vi "Begin.vi"() -> (0 "error out":errorcluster)   [LabVIEW 2012]
doc: "Called before other user functions, this VI is expected to open initial I/O refnums, load in file data, and do all program initialization. Notice that the <B>error out</B> terminal is simply used for data flow. Wiring it to other structures or subVIs ensures that this VI runs first."
uses:
  <vilib>/Rock Robotics/WPI/DriverStation/WPI_DriverStationRobotMode2.ctl
  <vilib>/Rock Robotics/WPI/CAN/Jaguar/SubVIs/WPI_CANJaguar_ControlMode.ctl
  <vilib>/Rock Robotics/WPI/CAN/Jaguar/SubVIs/WPI_CANJaguar_PositionReference.ctl
  <vilib>/Rock Robotics/WPI/CAN/Jaguar/SubVIs/WPI_CANJaguar_BrakeCoastMode.ctl
  <vilib>/Rock Robotics/WPI/SafetyOutput/WPI_SafetyOutputConfigMenu.ctl
  <vilib>/Rock Robotics/SystemInterfaces/DIO/FPGA_DIOChannel.ctl
  <vilib>/Rock Robotics/SystemInterfaces/DIO/FPGA_DIOPWMChannel.ctl
  <vilib>/Rock Robotics/WPI/CAN/Jaguar/SubVIs/WPI_CANJaguar_SpeedReference.ctl
  <vilib>/Rock Robotics/WPI/Joystick/WPI_JoystickDeviceEnum.ctl
  Robot Global Data.vi
  <vilib>/Rock Robotics/WPI/MotorControl/WPI_MotorControlOpenCANJaguar.vi
  <vilib>/Rock Robotics/WPI/MotorControl/WPI_MotorControlOpen Victor.vi
  <vilib>/Rock Robotics/WPI/RobotDrive/WPI_RobotDriveOpen4MotorWithExistingMotors.vi
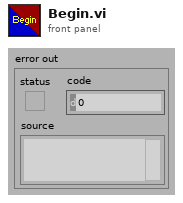
[diagram p1: front panel]
types:
  T1 = typedef "WPI_DriverStationRobotMode2.ctl" = enum16{"Autonomous Disabled", "Autonomous Enabled", "Teleop Disabled", "Teleop Enabled", "Timeout", "Finish", "Test Disabled", "Test Enabled"}
  T2 = typedef "WPI_CANJaguar_BrakeCoastMode.ctl" = enum8{"Jumper", "Brake", "Coast"}
  T3 = typedef "WPI_CANJaguar_ControlMode.ctl" = enum8{"Percent VBus", "Current", "Speed", "Position", "Voltage"}
  T4 = typedef "WPI_MotorControlDeviceRef.ctl" = cluster{"DeviceStatus":errorcluster, "Type":enum16{"PWM", "CAN"}, "PWM":cluster{"Digital Module":T5, "PWM Channel":T6, "DeadBand":T7}, "CAN":cluster{"Device Number":u8, "Control Mode":T3, "Semaphore":T8, "Max Vout":dbl}, "Invert":bool, "TransformRef":T9, "InvTransformRef":T9}
  T5 = typedef "FPGA_TypedefDigitalModule.ctl" = enum16{"Digital Module 1", "Digital Module 2"}
  T6 = typedef "FPGA_DIOPWMChannel.ctl" = enum8{"PWM 1", "PWM 2", "PWM 3", "PWM 4", "PWM 5", "PWM 6", "PWM 7", "PWM 8", "PWM 9", "PWM 10", "Invalid"}
  T7 = typedef "WPI_PWMDeadband.ctl" = cluster{"Name":string, "maxPositivePwm":i32, "minPositivePwm":i32, "centerPwm":i32, "maxNegativePwm":i32, "minNegativePwm":i32, "angularRange":u16}
  T8 = typedef "Semaphore RefNum" = refnum<k1>
  T9 = typedef "WPI_PWMTransform_ConPane.ctl" = refnum<vi>
  T10 = typedef "WPI_CANJaguar_SpeedReference.ctl" = u8
  T11 = typedef "WPI_RobotDriveDevRef.ctl" = cluster{"DevStatus":errorcluster, "Motors[]":T4[], "Square Inputs":bool, "Max Output":dbl, "Isochronous":bool}
  T12 = typedef "WPI_SafetyOutputConfigMenu.ctl" = enum16{"Enable", "Disable"}
  T13 = typedef "WPI_CANJaguar_PositionReference.ctl" = u8
  T14 = typedef "WPI_JoystickDeviceEnum.ctl" = enum16{"USB 1", "USB 2", "USB 3", "USB 4", "Kinect 1", "Kinect 2"}
  T15 = typedef "WPI_JoystickDevRef.ctl" = cluster{"Device":T14}
  T16 = typedef "FPGA_DIOChannel.ctl" = enum8{"DIO 1", "DIO 2", "DIO 3", "DIO 4", "DIO 5", "DIO 6", "DIO 7", "DIO 8", "DIO 9", "DIO 10", "DIO 11", "DIO 12", "DIO 13", "DIO 14", "Invalid"}
  T17 = typedef "WPI_DigitalInputDevRef.ctl" = cluster{"DevStatus":errorcluster, "DIO Channel":T16, "Digital Module":T5}
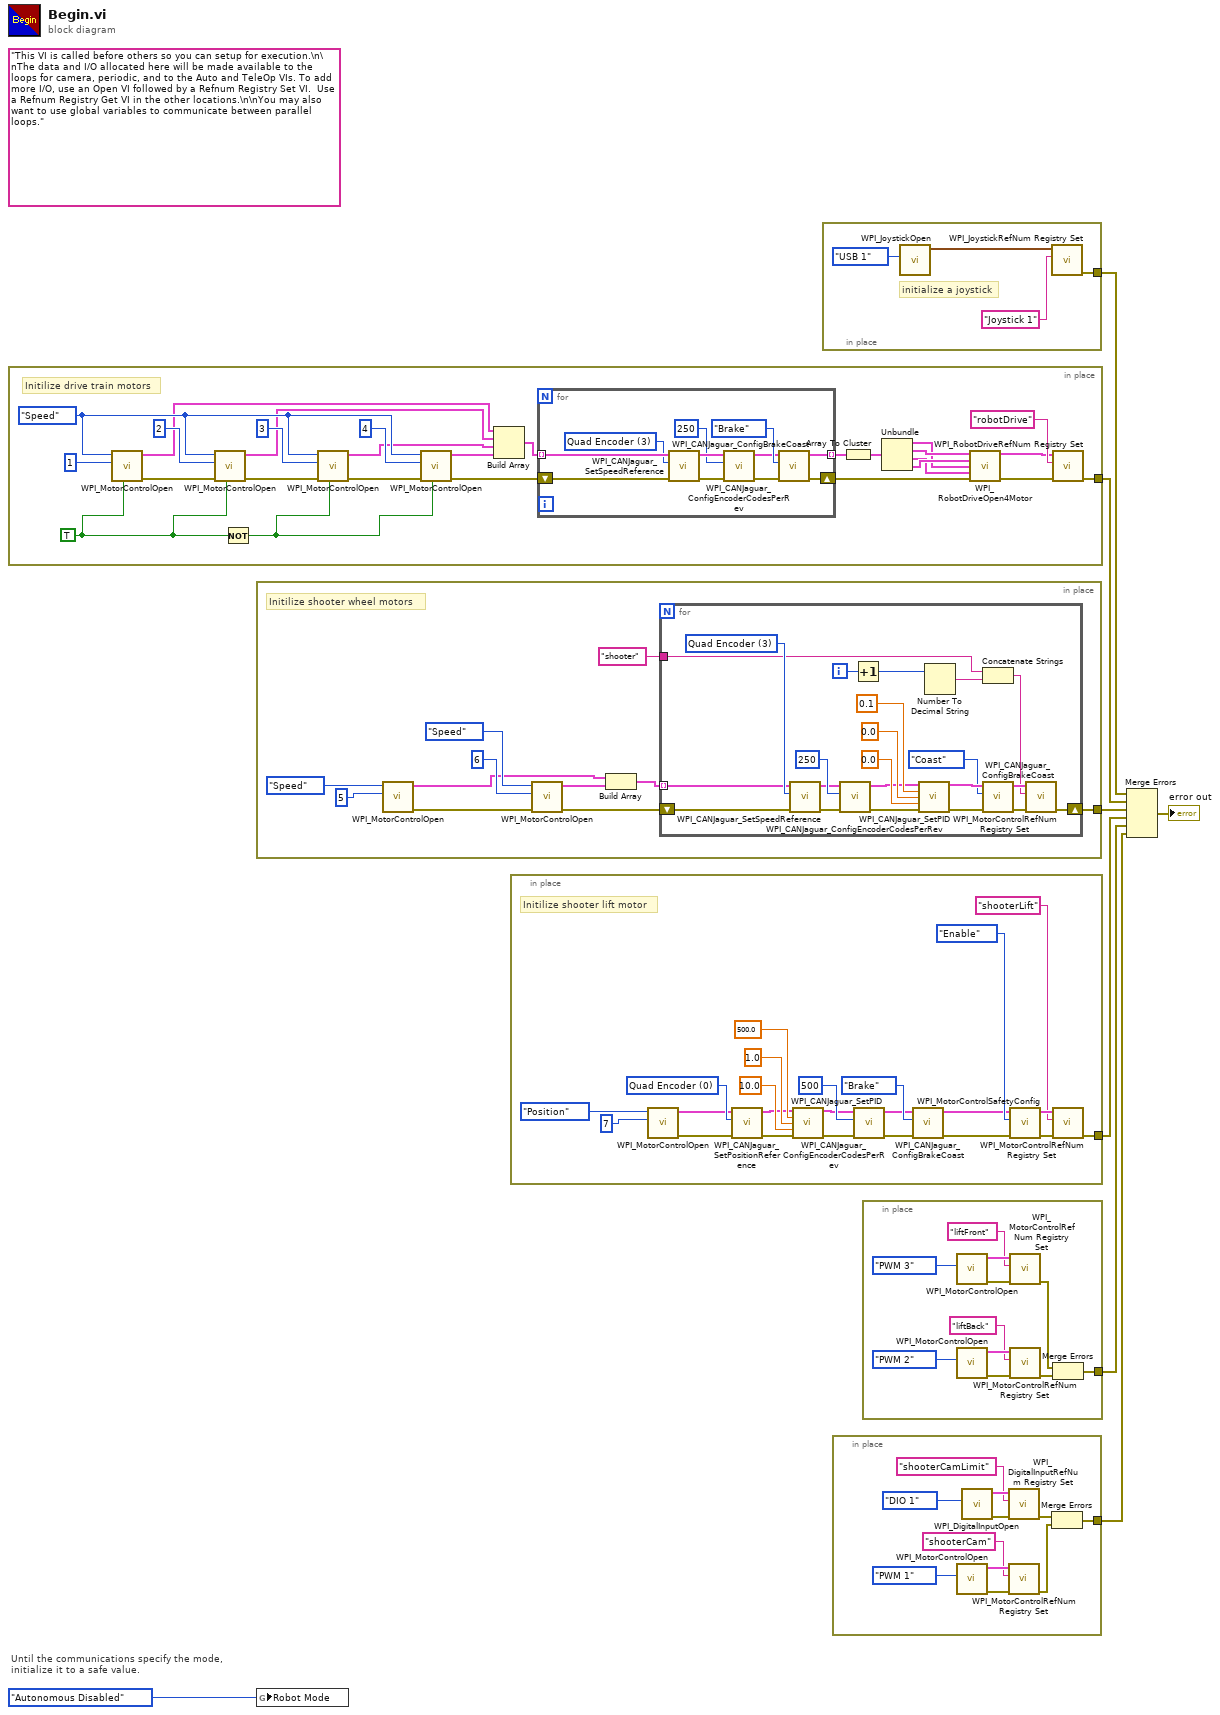
[diagram p0: block diagram]
diagram:
  (unwired) "This VI is called before others so you can setup for execution.\n\nThe data and I/O allocated here will be made available to the loops for camera, periodic, and to the Auto and TeleOp VIs. To add more I/O, use an Open VI followed by a Refnum Registry Set VI.  Use a Refnum Registry Get VI in the other locations.\n\nYou may also want to use global variables to communicate between parallel loops."
  # "Until the communications specify the mode,\ninitialize it to a safe value."
  n1 = in-place {
    in-place-border: [w35] -> w7
    w29 = TRUE ("Invert")
    w34 = WPI_CANJaguar_ControlMode."Speed" ("Control Mode")
    # "Initilize drive train motors"
    n2 = call-poly <vilib>:"WPI_MotorControlOpen.vi"("Invert"=w29, "Device Number"=u8 1, "Control Mode"=w34) -> ("error out"=w27:errorcluster, "MotorControlDeviceRef"=w24:T4)  [unwired: 7 in]
    n3 = call-poly <vilib>:"WPI_MotorControlOpen.vi"("Invert"=w29, "error in (no error)"=w27, "Device Number"=u8 2, "Control Mode"=w34) -> ("error out"=w26:errorcluster, "MotorControlDeviceRef"=w23:T4)  [unwired: 6 in]
    n4 = Not(x=w29) -> (.not. x?=w28:bool)
    n5 = call-poly <vilib>:"WPI_MotorControlOpen.vi"("Invert"=w28, "error in (no error)"=w26, "Device Number"=u8 3, "Control Mode"=w34) -> ("error out"=w25:errorcluster, "MotorControlDeviceRef"=w22:T4)  [unwired: 6 in]
    n6 = call-poly <vilib>:"WPI_MotorControlOpen.vi"("Invert"=w28, "error in (no error)"=w25, "Device Number"=u8 4, "Control Mode"=w34) -> ("error out"=w10:errorcluster, "MotorControlDeviceRef"=w21:T4)  [unwired: 6 in]
    n7 = Build Array(w24, w23, w22, w21) -> (w19:T4[])
    n8 = for {
      tunnel: w19 -> [w43] mode=indexing
      tunnel: [w45] -> w18 mode=indexing
      shift-right: [w44] -> w9
      shift-left: w10 -> [w42]
      w41 = T10 3 items=["Encoder"=0, "Inv Encoder"=2, "Quad Encoder"=3, "None"=255] ("Speed Reference")
      n9 = call <vilib>:"WPI_CANJaguar_SetSpeedReference.vi"("error in (no error)"=w42, "Speed Reference"=w41, "CAN Jaguar Ref"=w43) -> ("error out"=w40:errorcluster, "CAN Jaguar Ref Out"=w39:T4)  [unwired: 7 in]
      n10 = call <vilib>:"WPI_CANJaguar_ConfigEncoderCodesPerRev.vi"("error in (no error)"=w40, "Encoder Codes Per Rev"=u16 250, "CAN Jaguar Ref"=w39) -> ("error out"=w36:errorcluster, "CAN Jaguar Ref Out"=w37:T4)  [unwired: 7 in]
      n11 = call <vilib>:"WPI_CANJaguar_ConfigBrakeCoast.vi"("error in (no error)"=w36, "Brake / Coast Mode"=WPI_CANJaguar_BrakeCoastMode."Brake", "CAN Jaguar Ref"=w37) -> ("error out"=w44:errorcluster, "CAN Jaguar Ref Out"=w45:T4)  [unwired: 7 in]
    }
    n12 = Array To Cluster(array=w18) -> (cluster=w17:cluster{"[0]":T4, "[1]":T4, "[2]":T4, "[3]":T4})
    n13 = Unbundle(w17) -> ("[0]"=w11:T4, "[1]"=w12:T4, "[2]"=w13:T4, "[3]"=w14:T4)
    n14 = call-poly <vilib>:"WPI_RobotDriveOpen4Motor.vi"("Rear Left Motor Dev Ref"=w12, "Rear Right Motor Dev Ref"=w14, "Front Left Motor Dev Ref"=w11, "Front Right Motor Dev Ref"=w13, "error in (no error)"=w9) -> ("RobotDriveDevRef"=w15:T11, "error out"=w16:errorcluster)  [unwired: 9 in]
    n15 = call <vilib>:"WPI_RobotDriveRefNum Registry Set.vi"("error in (no error)"=w16, "refnum name"="robotDrive", "RobotDriveDevRef"=w15) -> ("error out"=w35:errorcluster)  [unwired: 7 in, 1 out]
  }
  n16 = in-place {
    in-place-border: [w57] -> w6
    # "Initilize shooter wheel motors"
    n17 = call-poly <vilib>:"WPI_MotorControlOpen.vi"("Device Number"=u8 5, "Control Mode"=WPI_CANJaguar_ControlMode."Speed") -> ("error out"=w52:errorcluster, "MotorControlDeviceRef"=w50:T4)  [unwired: 8 in]
    n18 = call-poly <vilib>:"WPI_MotorControlOpen.vi"("error in (no error)"=w52, "Device Number"=u8 6, "Control Mode"=WPI_CANJaguar_ControlMode."Speed") -> ("error out"=w48:errorcluster, "MotorControlDeviceRef"=w51:T4)  [unwired: 7 in]
    n19 = Build Array(w50, w51) -> (w49:T4[])
    n20 = for {
      tunnel: w49 -> [w68] mode=indexing
      tunnel: "shooter" -> [w62]
      shift-right: [w59] -> w57
      shift-left: w48 -> [w67]
      i -> [w66]
      w69 = T10 3 items=["Encoder"=0, "Inv Encoder"=2, "Quad Encoder"=3, "None"=255] ("Speed Reference")
      n21 = call <vilib>:"WPI_CANJaguar_SetSpeedReference.vi"("error in (no error)"=w67, "Speed Reference"=w69, "CAN Jaguar Ref"=w68) -> ("error out"=w70:errorcluster, "CAN Jaguar Ref Out"=w71:T4)  [unwired: 7 in]
      n22 = call <vilib>:"WPI_CANJaguar_ConfigEncoderCodesPerRev.vi"("error in (no error)"=w70, "Encoder Codes Per Rev"=u16 250, "CAN Jaguar Ref"=w71) -> ("error out"=w74:errorcluster, "CAN Jaguar Ref Out"=w73:T4)  [unwired: 7 in]
      n23 = Increment(x=w66) -> (x+1=w65:i32)
      n24 = call <vilib>:"WPI_CANJaguar_SetPID.vi"("CAN Jaguar Ref"=w73, "P"=0.1, "I"=0.0, "D"=0.0, "error in (no error)"=w74) -> ("CAN Jaguar Ref Out"=w75:T4, "error out"=w76:errorcluster)  [unwired: 9 in]
      n25 = Number To Decimal String(number=w65) -> (decimal integer string=w61:string)  [unwired: 1 in]
      n26 = Concatenate Strings(w62, w61) -> (w60:string)
      n27 = call <vilib>:"WPI_CANJaguar_ConfigBrakeCoast.vi"("error in (no error)"=w76, "Brake / Coast Mode"=WPI_CANJaguar_BrakeCoastMode."Coast", "CAN Jaguar Ref"=w75) -> ("error out"=w64:errorcluster, "CAN Jaguar Ref Out"=w63:T4)  [unwired: 7 in]
      n28 = call <vilib>:"WPI_MotorControlRefNum Registry Set.vi"("error in (no error)"=w64, "refnum name"=w60, "MotorControlDevRef"=w63) -> ("error out"=w59:errorcluster)  [unwired: 7 in, 1 out]
    }
  }
  n29 = global write "Robot Global Data.vi" "Robot Mode"(WPI_DriverStationRobotMode2."Autonomous Disabled" ("Robot Mode")) -> ()
  n30 = in-place {
    in-place-border: [w102] -> w3
    w88 = T13 0 items=["Quad Encoder"=0, "Potentiometer"=1, "None"=255] ("Position Reference")
    # "Initilize shooter lift motor"
    n31 = call-poly <vilib>:"WPI_MotorControlOpen.vi"("Device Number"=u8 7, "Control Mode"=WPI_CANJaguar_ControlMode."Position") -> ("error out"=w86:errorcluster, "MotorControlDeviceRef"=w87:T4)  [unwired: 8 in]
    n32 = call <vilib>:"WPI_CANJaguar_SetPositionReference.vi"("error in (no error)"=w86, "Position Reference"=w88, "CAN Jaguar Ref"=w87) -> ("error out"=w90:errorcluster, "CAN Jaguar Ref Out"=w89:T4)  [unwired: 7 in]
    n33 = call <vilib>:"WPI_CANJaguar_SetPID.vi"("CAN Jaguar Ref"=w89, "P"=500.0, "I"=1.0, "D"=10.0, "error in (no error)"=w90) -> ("CAN Jaguar Ref Out"=w95:T4, "error out"=w94:errorcluster)  [unwired: 9 in]
    n34 = call <vilib>:"WPI_CANJaguar_ConfigEncoderCodesPerRev.vi"("error in (no error)"=w94, "Encoder Codes Per Rev"=u16 500, "CAN Jaguar Ref"=w95) -> ("error out"=w97:errorcluster, "CAN Jaguar Ref Out"=w98:T4)  [unwired: 7 in]
    n35 = call <vilib>:"WPI_CANJaguar_ConfigBrakeCoast.vi"("error in (no error)"=w97, "Brake / Coast Mode"=WPI_CANJaguar_BrakeCoastMode."Brake", "CAN Jaguar Ref"=w98) -> ("error out"=w80:errorcluster, "CAN Jaguar Ref Out"=w81:T4)  [unwired: 7 in]
    n36 = call <vilib>:"WPI_MotorControlSafetyConfig.vi"("error in (no error)"=w80, "mode"=WPI_SafetyOutputConfigMenu."Enable", "MotorControlDevRef"=w81) -> ("error out"=w100:errorcluster, "MotorControlDevRef"=w101:T4)  [unwired: 7 in]
    n37 = call <vilib>:"WPI_MotorControlRefNum Registry Set.vi"("error in (no error)"=w100, "refnum name"="shooterLift", "MotorControlDevRef"=w101) -> ("error out"=w102:errorcluster)  [unwired: 7 in, 1 out]
  }
  n38 = in-place {
    in-place-border: [w103] -> w4
    # "initialize a joystick"
    n39 = call <vilib>:"WPI_JoystickOpen.vi"("JoystickDevice"=WPI_JoystickDeviceEnum."USB 1") -> ("JoystickDevRef"=w105:T15)  [unwired: 10 in]
    n40 = call <vilib>:"WPI_JoystickRefNum Registry Set.vi"("refnum name"="Joystick 1", "JoystickDevRef"=w105) -> ("error out"=w103:errorcluster)  [unwired: 8 in, 1 out]
  }
  n41 = in-place {
    in-place-border: [w117] -> w1
    n42 = call-poly <vilib>:"WPI_MotorControlOpen.vi"("PWM Channel"=FPGA_DIOPWMChannel."PWM 1") -> ("error out"=w110:errorcluster, "MotorControlDeviceRef"=w111:T4)  [unwired: 9 in]
    n43 = call <vilib>:"WPI_DigitalInputOpen.vi"("DIO Channel"=FPGA_DIOChannel."DIO 1") -> ("error out"=w115:errorcluster, "DigitalInputDevRef"=w114:T17)  [unwired: 9 in]
    n44 = call <vilib>:"WPI_DigitalInputRefNum Registry Set.vi"("error in (no error)"=w115, "refnum name"="shooterCamLimit", "DigitalInputDevRef"=w114) -> ("error out"=w108:errorcluster)  [unwired: 7 in, 1 out]
    n45 = call <vilib>:"WPI_MotorControlRefNum Registry Set.vi"("error in (no error)"=w110, "refnum name"="shooterCam", "MotorControlDevRef"=w111) -> ("error out"=w107:errorcluster)  [unwired: 7 in, 1 out]
    n46 = Merge Errors(w108, w107) -> (w117:errorcluster)
  }
  n47 = in-place {
    in-place-border: [w128] -> w2
    n48 = call-poly <vilib>:"WPI_MotorControlOpen.vi"("PWM Channel"=FPGA_DIOPWMChannel."PWM 3") -> ("error out"=w125:errorcluster, "MotorControlDeviceRef"=w124:T4)  [unwired: 9 in]
    n49 = call-poly <vilib>:"WPI_MotorControlOpen.vi"("PWM Channel"=FPGA_DIOPWMChannel."PWM 2") -> ("error out"=w122:errorcluster, "MotorControlDeviceRef"=w121:T4)  [unwired: 9 in]
    n50 = call <vilib>:"WPI_MotorControlRefNum Registry Set.vi"("error in (no error)"=w125, "refnum name"="liftFront", "MotorControlDevRef"=w124) -> ("error out"=w119:errorcluster)  [unwired: 7 in, 1 out]
    n51 = call <vilib>:"WPI_MotorControlRefNum Registry Set.vi"("error in (no error)"=w122, "refnum name"="liftBack", "MotorControlDevRef"=w121) -> ("error out"=w118:errorcluster)  [unwired: 7 in, 1 out]
    n52 = Merge Errors(w119, w118) -> (w128:errorcluster)
  }
  n53 = Merge Errors(w4, w7, w6, w3, w2, w1) -> (→"error out":errorcluster)
